vi "科盛查询命令解析.vi"(10 "解析参数选择":enum16{"查询采样记录", "查询瓶记录", "查询系统状态"}(ring), 11 "命令输入":string) -> (3 "Variant":variant)   [LabVIEW 2016, in "科盛超标留样.lvlib"]
panel:
  out "查询系统状态":T1
  out "查询瓶记录":T2
  out "输出数组":T3(array[cluster])
  out "查询采样记录":T4
  out "数组":string[](array[string])
  # "1506 0610 1101 0101 0102 0100 0200 0102 1506 0610 1101 0101 1506 0610 1101 0101 0102 0100 0200 0102 1506 0610 1101 0101"
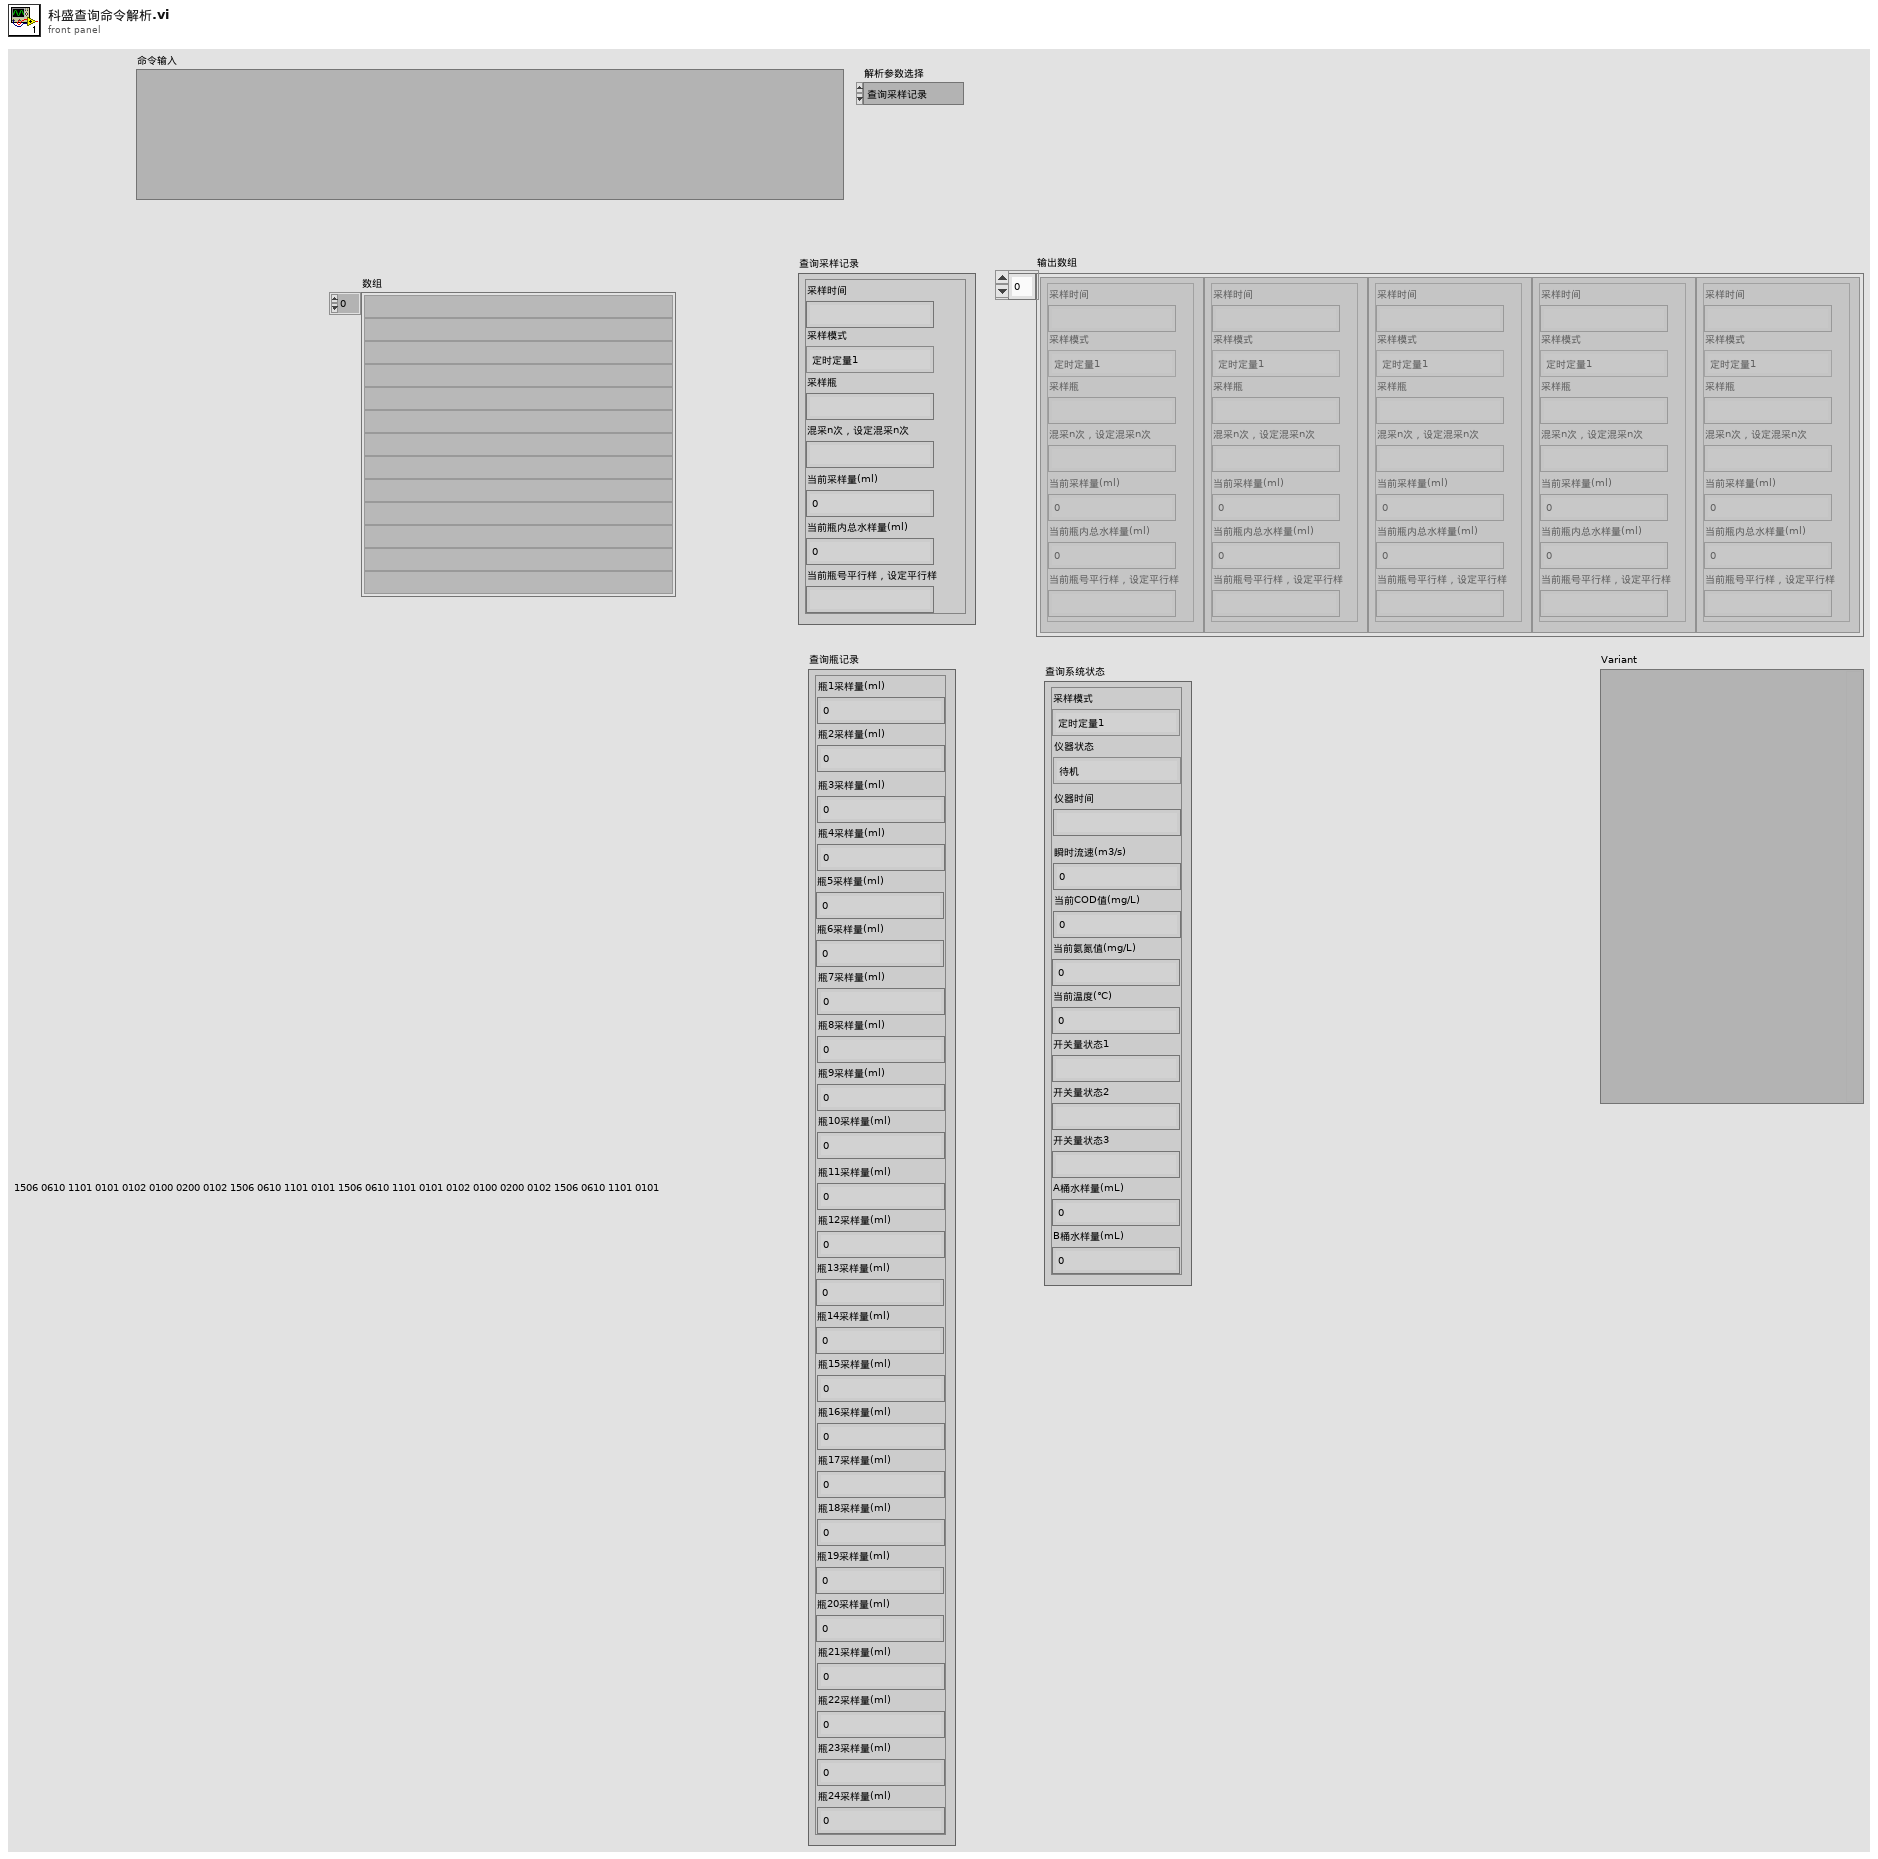
[diagram p1: front panel]
types:
  T1 = cluster{"采样模式":enum16{"定时定量1", "定时定量2", "定流定量", "定时比例", "同步留样", "超标留样", "触发采样", "定时采样1", "定流供样", "定时采样2", "远程取样", "手动取样", "流量跟踪"}, "仪器状态":enum16{"待机", "运行中"}, "仪器时间":string, "瞬时流速(m3/s)":dbl, "当前COD值(mg/L)":dbl, "当前氨氮值(mg/L)":dbl, "当前温度(℃)":dbl, "开关量状态1":string, "开关量状态2":string, "开关量状态3":string, "A桶水样量(mL)":dbl, "B桶水样量(mL)":dbl}
  T2 = cluster{"瓶1采样量(ml)":dbl, "瓶2采样量(ml)":dbl, "瓶3采样量(ml)":dbl, "瓶4采样量(ml)":dbl, "瓶5采样量(ml)":dbl, "瓶6采样量(ml)":dbl, "瓶7采样量(ml)":dbl, "瓶8采样量(ml)":dbl, "瓶9采样量(ml)":dbl, "瓶10采样量(ml)":dbl, "瓶11采样量(ml)":dbl, "瓶12采样量(ml)":dbl, "瓶13采样量(ml)":dbl, "瓶14采样量(ml)":dbl, "瓶15采样量(ml)":dbl, "瓶16采样量(ml)":dbl, "瓶17采样量(ml)":dbl, "瓶18采样量(ml)":dbl, "瓶19采样量(ml)":dbl, "瓶20采样量(ml)":dbl, "瓶21采样量(ml)":dbl, "瓶22采样量(ml)":dbl, "瓶23采样量(ml)":dbl, "瓶24采样量(ml)":dbl}
  T3 = cluster{"采样时间":string, "采样模式":enum16{"定时定量1", "定时定量2", "定流定量", "定时比例", "同步留样", "超标留样", "触发采样", "定时采样1", "定流供样", "定时采样2", "远程取样", "手动取样", "流量跟踪"}, "采样瓶":string, "混采n次，设定混采n次":string, "当前采样量(ml)":dbl, "当前瓶内总水样量(ml)":dbl, "当前瓶号平行样，设定平行样":string}[]
  T4 = cluster{"采样时间":string, "采样模式":enum16{"定时定量1", "定时定量2", "定流定量", "定时比例", "同步留样", "超标留样", "触发采样", "定时采样1", "定流供样", "定时采样2", "远程取样", "手动取样", "流量跟踪"}, "采样瓶":string, "混采n次，设定混采n次":string, "当前采样量(ml)":dbl, "当前瓶内总水样量(ml)":dbl, "当前瓶号平行样，设定平行样":string}
  T5 = cluster{"[0]":i32, "[1]":i32, "[2]":i32, "[3]":i32, "[4]":i32, "[5]":i32, "[6]":i32, "[7]":i32, "[8]":i32, "[9]":i32, "[10]":i32, "[11]":i32, "[12]":i32, "[13]":i32, "[14]":i32, "[15]":i32, "[16]":i32, "[17]":i32, "[18]":i32, "[19]":i32, "[20]":i32, "[21]":i32, "[22]":i32, "[23]":i32}
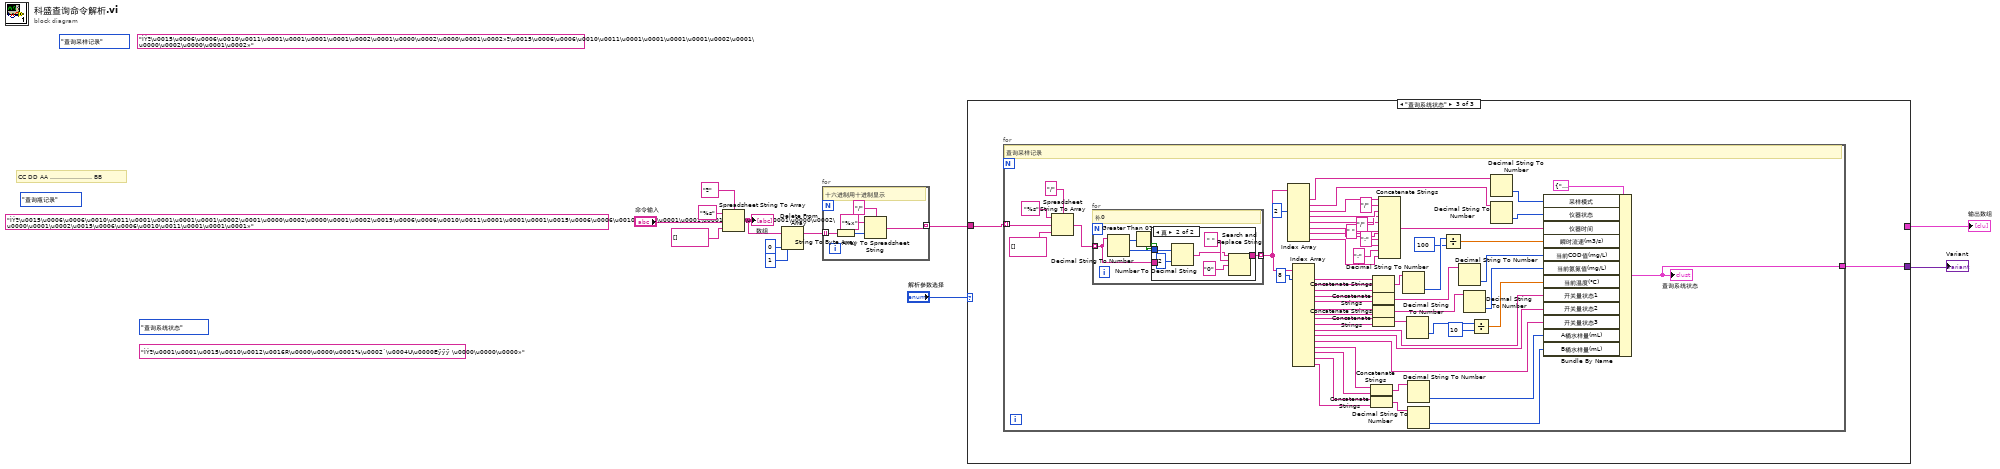
[diagram p0: block diagram]
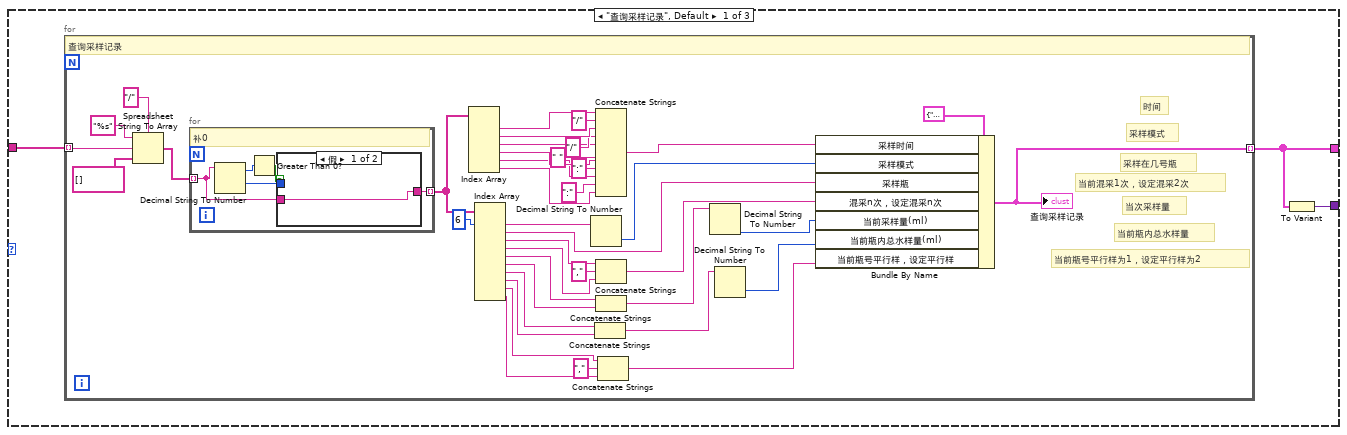
[diagram p2: hidden frame]
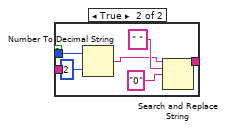
[diagram p3: hidden frame]
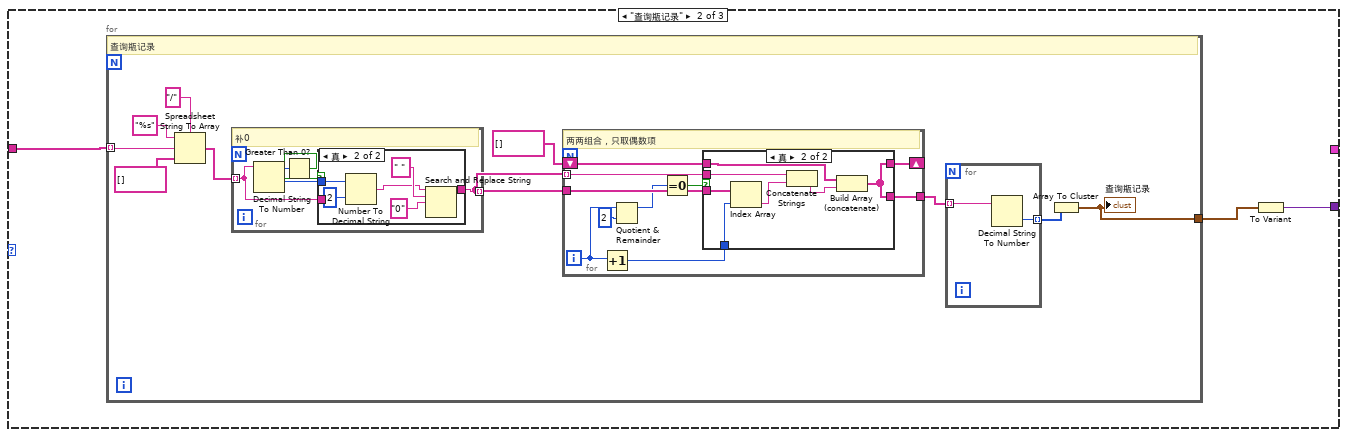
[diagram p4: hidden frame]
diagram:
  (unwired) enum16{"查询采样记录", "查询瓶记录", "查询系统状态"}."查询系统状态"
  (unwired) "ÌÝª\u0001\u0001\u0015\u0010\u0012\u0016R\u0000\u0000\u0001%\u0002`\u0004U\u0000Eÿÿÿ \u0000\u0000\u0000»"
  (unwired) enum16{"查询采样记录", "查询瓶记录", "查询系统状态"}."查询瓶记录"
  (unwired) "ÌÝª\u0015\u0006\u0006\u0010\u0011\u0001\u0001\u0001\u0001\u0002\u0001\u0000\u0002\u0000\u0001\u0002\u0015\u0006\u0006\u0010\u0011\u0001\u0001\u0001\u0015\u0006\u0006\u0010\u0011\u0001\u0001\u0001\u0001\u0002\u0001\u0000\u0002\u0000\u0001\u0002\u0015\u0006\u0006\u0010\u0011\u0001\u0001\u0001»"
  (unwired) enum16{"查询采样记录", "查询瓶记录", "查询系统状态"}."查询采样记录"
  (unwired) "ÌÝª\u0015\u0006\u0006\u0010\u0011\u0001\u0001\u0001\u0001\u0002\u0001\u0000\u0002\u0000\u0001\u0002»ª\u0015\u0006\u0006\u0010\u0011\u0001\u0001\u0001\u0001\u0002\u0001\u0000\u0002\u0000\u0001\u0002»"
  # "CC DD AA ………………… BB"
  n1 = Spreadsheet String To Array(delimiter (Tab)="ª" ("分隔符(Tab)"), format string="%s" ("格式字符串"), spreadsheet string="命令输入", array type (2D Dbl)=string[] []) -> (array=w9:string[])
  "数组" <- w9
  n2 = Delete From Array(array=w9, length=1 ("长度"), index=0 ("索引")) -> (array with subset deleted=w6:string[])  [unwired: 1 out]
  n3 = for "For循环" {
    tunnel: w6 -> [w15] mode=indexing
    tunnel: [w13] -> w5 mode=indexing
    # "十六进制用十进制显示"
    n4 = String To Byte Array(string=w15) -> (unsigned byte array=w16:u8[])
    n5 = Array To Spreadsheet String(delimiter (Tab)="/" ("分隔符(Tab)"), array=w16, 3:"%x" ("格式字符串")) -> (spreadsheet string=w13:string)
  }
  n6 = case shown="\"查询系统状态\"" "解析参数选择" {
    tunnel: w5 -> [w20 w75 w119]
    tunnel: [w19 _ _] -> w4
    tunnel: [w18 w73 w118] -> w1
    frame "查询采样记录", Default {
      n7 = for {
        tunnel: w20 -> [w58] mode=indexing
        tunnel: [w21] -> w19 mode=indexing
        # "当前瓶号平行样为1，设定平行样为2"
        # "当前瓶内总水样量"
        # "当次采样量"
        # "当前混采1次，设定混采2次"
        # "采样在几号瓶"
        # "采样模式"
        # "时间"
        # "查询采样记录"
        n8 = Spreadsheet String To Array(delimiter (Tab)="/" ("分隔符(Tab)"), format string="%s" ("格式字符串"), spreadsheet string=w58, array type (2D Dbl)=string[] []) -> (array=w45:string[])
        n9 = for {
          tunnel: w45 -> [w61] mode=indexing
          tunnel: [w64] -> w40 mode=indexing
          # "补0"
          n10 = Decimal String To Number(string=w61) -> (offset past number=w63:i32, number=w65:i32)  [unwired: 2 in]
          n11 = Greater Than 0?(x=w63) -> (x > 0?=w62:bool)
          n12 = case shown="假" w62 {
            tunnel: w65 -> [_ w68]
            tunnel: [w66 w67] -> w64
            tunnel: w61 -> [w66 _]
            frame False {
            }
            frame True {
              n13 = Number To Decimal String(number=w68, width (-)=i16 2 ("宽度(-)")) -> (decimal integer string=w70:string)
              n14 = Search and Replace String(input string=w70, search string=" " ("搜索字符串"), replace string="0" ("替换字符串(\"\")")) -> (result string=w67:string)  [unwired: 5 in, 3 out]
            }
          }
        }
        n15 = Index Array(array=w40) -> (element #1=w56:string, element #2=w54:string, element #3=w52:string, element #4=w50:string, element #5=w48:string, element #6=w46:string)  [unwired: 6 in]
        n16 = Index Array(array=w40, index #1=6 ("索引")) -> (element #1=w42:string, element #2=w39:string, element #3=w38:string, element #4=w36:string, element #5=w34:string, element #6=w33:string, element #7=w32:string, element #8=w31:string, element #9=w29:string, element #10=w28:string)  [unwired: 9 in]
        n17 = Decimal String To Number(string=w42) -> (number=w41:i32)  [unwired: 2 in, 1 out]
        n18 = Concatenate Strings(w32, w31) -> (w24:string)
        n19 = Concatenate Strings(w56, "/" ("字符串"), w54, "/" ("字符串"), w52, " " ("字符串"), w50, ":" ("字符串"), w48, ":" ("字符串"), w46) -> (w44:string)
        n20 = Concatenate Strings(w38, "," ("字符串"), w36) -> (w35:string)
        n21 = Concatenate Strings(w34, w33) -> (w25:string)
        n22 = Concatenate Strings(w29, "," ("字符串"), w28) -> (w27:string)
        n23 = Decimal String To Number(string=w25) -> (number=w23:i32)  [unwired: 2 in, 1 out]
        n24 = Decimal String To Number(string=w24) -> (number=w22:i32)  [unwired: 2 in, 1 out]
        n25 = Bundle By Name(cluster=T4 {"采样时间"="", "采样模式"=enum."定时定量1", "采样瓶"="", "混采n次，设定混采n次"="", "当前采样量(ml)"=0.0, "当前瓶内总水样量(ml)"=0.0, "当前瓶号平行样，设定平行样"=""} ("簇"), "采样时间"=w44, "采样模式"=w41, "采样瓶"=w39, "混采n次，设定混采n次"=w35, "当前采样量(ml)"=w23, "当前瓶内总水样量(ml)"=w22, "当前瓶号平行样，设定平行样"=w27) -> (w21:T4)
        "查询采样记录" <- w21
      }
      n26 = To Variant(anything=w19) -> (Variant=w18:variant)
    }
    frame "查询瓶记录" {
      n27 = for {
        tunnel: w75 -> [w83] mode=indexing
        tunnel: [w76] -> w74
        # "查询瓶记录"
        n28 = Spreadsheet String To Array(delimiter (Tab)="/" ("分隔符(Tab)"), format string="%s" ("格式字符串"), spreadsheet string=w83, array type (2D Dbl)=string[] []) -> (array=w81:string[])
        n29 = for {
          tunnel: w81 -> [w106] mode=indexing
          tunnel: [w109] -> w80 mode=indexing
          # "补0"
          n30 = Decimal String To Number(string=w106) -> (offset past number=w108:i32, number=w110:i32)  [unwired: 2 in]
          n31 = Greater Than 0?(x=w108) -> (x > 0?=w107:bool)
          n32 = case shown="真" w107 {
            tunnel: w110 -> [_ w113]
            tunnel: [w111 w112] -> w109
            tunnel: w106 -> [w111 _]
            frame False {
            }
            frame True {
              n33 = Number To Decimal String(number=w113, width (-)=i16 2 ("宽度(-)")) -> (decimal integer string=w115:string)
              n34 = Search and Replace String(input string=w115, search string=" " ("搜索字符串"), replace string="0" ("替换字符串(\"\")")) -> (result string=w112:string)  [unwired: 5 in, 3 out]
            }
          }
        }
        n35 = for {
          tunnel: w80 -> [w96]
          tunnel: w80 -> [w97] mode=indexing
          shift-right: [w88] -> _
          shift-left: string[] [] -> [w90]
          tunnel: [w89] -> w77
          i -> [w94]
          # "两两组合，只取偶数项"
          n36 = Increment(x=w94) -> (x+1=w95:i32)
          n37 = Quotient & Remainder(x=w94, y=2) -> (x-y*floor(x/y)=w92:i32)  [unwired: 1 out]
          n38 = Equal To 0?(x=w92) -> (x = 0?=w91:bool)
          n39 = case shown="真" w91 {
            tunnel: w97 -> [_ w105]
            tunnel: w96 -> [_ w104]
            tunnel: w95 -> [_ w103]
            tunnel: w90 -> [w98 w101]
            tunnel: [w98 w99] -> w89
            tunnel: [w98 w99] -> w88
            frame False {
            }
            frame True {
              n40 = Index Array(array=w104, index=w103) -> (element=w102:string)
              n41 = Concatenate Strings(w105, w102) -> (w100:string)
              n42 = Build Array (concatenate)(w101, w100) -> (w99:string[])
            }
          }
        }
        n43 = for {
          tunnel: w77 -> [w87] mode=indexing
          tunnel: [w86] -> w79 mode=indexing
          n44 = Decimal String To Number(string=w87) -> (number=w86:i32)  [unwired: 2 in, 1 out]
        }
        n45 = Array To Cluster(array=w79) -> (cluster=w76:T5)
        "查询瓶记录" <- w76
      }
      n46 = To Variant(anything=w74) -> (Variant=w73:variant)
    }
    frame "查询系统状态" {
      n47 = for {
        tunnel: w119 -> [w175] mode=indexing
        tunnel: [w120] -> w118
        # "查询采样记录"
        n48 = Spreadsheet String To Array(delimiter (Tab)="/" ("分隔符(Tab)"), format string="%s" ("格式字符串"), spreadsheet string=w175, array type (2D Dbl)=string[] []) -> (array=w162:string[])
        n49 = for {
          tunnel: w162 -> [w178] mode=indexing
          tunnel: [w181] -> w160 mode=indexing
          # "补0"
          n50 = Decimal String To Number(string=w178) -> (offset past number=w180:i32, number=w182:i32)  [unwired: 2 in]
          n51 = Greater Than 0?(x=w180) -> (x > 0?=w179:bool)
          n52 = case shown="真" w179 {
            tunnel: w182 -> [_ w185]
            tunnel: [w183 w184] -> w181
            tunnel: w178 -> [w183 _]
            frame False {
            }
            frame True {
              n53 = Number To Decimal String(number=w185, width (-)=i16 2 ("宽度(-)")) -> (decimal integer string=w187:string)
              n54 = Search and Replace String(input string=w187, search string=" " ("搜索字符串"), replace string="0" ("替换字符串(\"\")")) -> (result string=w184:string)  [unwired: 5 in, 3 out]
            }
          }
        }
        n55 = Index Array(array=w160, index #3=2 ("索引")) -> (element #1=w155:string, element #2=w154:string, element #3=w173:string, element #4=w171:string, element #5=w169:string, element #6=w167:string, element #7=w165:string, element #8=w163:string)  [unwired: 7 in]
        n56 = Index Array(array=w160, index #1=8 ("索引")) -> (element #1=w151:string, element #2=w150:string, element #3=w149:string, element #4=w144:string, element #5=w143:string, element #6=w141:string, element #7=w140:string, element #8=w137:string, element #9=w136:string, element #10=w123:string, element #11=w122:string, element #12=w121:string, element #13=w131:string, element #14=w130:string, element #15=w129:string, element #16=w128:string)  [unwired: 15 in]
        n57 = Concatenate Strings(w129, w128) -> (w126:string)
        n58 = Concatenate Strings(w131, w130) -> (w127:string)
        n59 = Concatenate Strings(w151, w150, w149) -> (w148:string)
        n60 = Concatenate Strings(w144, w143) -> (w138:string)
        n61 = Concatenate Strings(w141, w140) -> (w159:string)
        n62 = Concatenate Strings(w137, w136) -> (w134:string)
        n63 = Concatenate Strings(w173, "/" ("字符串"), w171, "/" ("字符串"), w169, " " ("字符串"), w167, ":" ("字符串"), w165, ":" ("字符串"), w163) -> (w156:string)
        n64 = Decimal String To Number(string=w148) -> (number=w147:i32)  [unwired: 2 in, 1 out]
        n65 = Decimal String To Number(string=w134) -> (number=w133:i32)  [unwired: 2 in, 1 out]
        n66 = Decimal String To Number(string=w127) -> (number=w125:i32)  [unwired: 2 in, 1 out]
        n67 = Decimal String To Number(string=w126) -> (number=w124:i32)  [unwired: 2 in, 1 out]
        n68 = Divide(x=w147, y=100) -> (x/y=w145:dbl)
        n69 = Decimal String To Number(string=w138) -> (number=w142:i32)  [unwired: 2 in, 1 out]
        n70 = Decimal String To Number(string=w159) -> (number=w139:i32)  [unwired: 2 in, 1 out]
        n71 = Divide(x=w133, y=10) -> (x/y=w132:dbl)
        n72 = Decimal String To Number(string=w154) -> (number=w153:i32)  [unwired: 2 in, 1 out]
        n73 = Decimal String To Number(string=w155) -> (number=w152:i32)  [unwired: 2 in, 1 out]
        n74 = Bundle By Name(cluster=T1 {"采样模式"=enum."定时定量1", "仪器状态"=enum."待机", "仪器时间"="", "瞬时流速(m3/s)"=0.0, "当前COD值(mg/L)"=0.0, "当前氨氮值(mg/L)"=0.0, "当前温度(℃)"=0.0, "开关量状态1"="", "开关量状态2"="", "开关量状态3"="", "A桶水样量(mL)"=0.0, "B桶水样量(mL)"=0.0} ("查询系统状态"), "采样模式"=w152, "仪器状态"=w153, "仪器时间"=w156, "瞬时流速(m3/s)"=w145, "当前COD值(mg/L)"=w142, "当前氨氮值(mg/L)"=w139, "当前温度(℃)"=w132, "开关量状态1"=w123, "开关量状态2"=w122, "开关量状态3"=w121, "A桶水样量(mL)"=w125, "B桶水样量(mL)"=w124) -> (w120:T1)
        "查询系统状态" <- w120
      }
    }
  }
  "输出数组" <- w4
  "Variant" <- w1
